vi "Wait Until Not Busy.vi"(6 "chip select  (1st chip)":enum16{"1st chip", "2nd chip"}(ring), 8 "error in (no error)":errorcluster, 11 "LCD in":u32) -> (0 "error out":errorcluster, 3 "LCD out":u32)   [LabVIEW 2015, in "HD44780 FPGA.lvlib"]
uses:
  <vilib>/EmbeddedDisplay/Hitachi HD44780/FPGA/HD44780 FPGA.lvlib
  <vilib>/EmbeddedDisplay/Hitachi HD44780/Common/HD44780 Common.lvlib
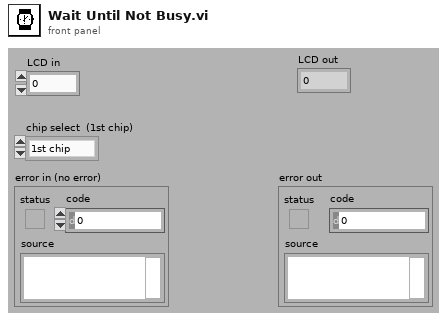
[diagram p1: front panel]
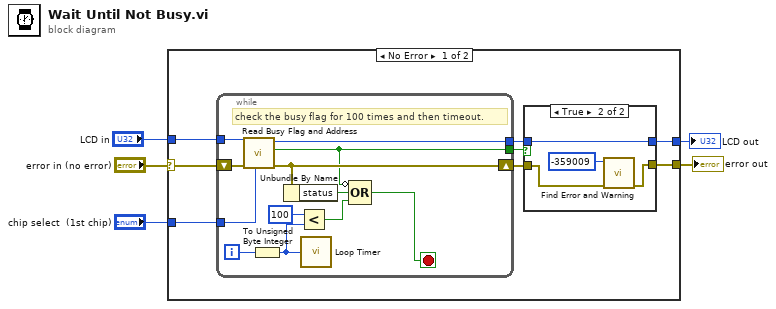
[diagram p0: block diagram]
diagram:
  n1 = case shown="No Error" "error in (no error)" {
    selector: "error in (no error)" -> [w9 w33]
    tunnel: [w12 w33] -> w4
    tunnel: "chip select  (1st chip)" -> [w10 _]
    tunnel: "LCD in" -> [w8 w32]
    tunnel: [w7 w32] -> w1
    frame No Error {
      n2 = while {
        shift-right: [w23] -> w11
        shift-left: w9 -> [w24]
        tunnel: w10 -> [w14]
        tunnel: [w22] -> w13
        tunnel: w8 -> [w21]
        tunnel: [w20] -> w6
        i -> [w18]
        stop <- w19 stop-if-true
        # "check the busy flag for 100 times and then timeout."
        n3 = call <vilib>:"Read Busy Flag and Address.vi"("chip select (1st chip)"=w14, "error in (no error)"=w24, "LCD in"=w21) -> ("error out"=w23:errorcluster, "busy flag"=w22:bool, "LCD out"=w20:u32)  [unwired: 5 in, 1 out]
        n4 = To Unsigned Byte Integer(number=w18) -> (unsigned 8bit integer=w15:u8)
        n5 = Unbundle By Name(w23) -> ("status"=w25:bool)
        n6 = Less?(x=u8 100, y=w15) -> (x < y?=w16:bool)
        n7 = call "Loop Timer"("Count(mSec)"=w15) -> ()  [unwired: 1 out]
        n8 = Compound Arithmetic op=OR(invert w22, w25, w16) -> (w19:bool)
      }
      n9 = case shown="True" w13 {
        tunnel: [w27 w28] -> w12
        tunnel: w11 -> [w27 w29]
        tunnel: [w26 w31] -> w7
        tunnel: w6 -> [w26 w31]
        frame False {
        }
        frame True {
          n10 = call <vilib>:"Find Error and Warning.vi"("error in (no error)"=w29, "error code"=-359009) -> ("error out"=w28:errorcluster)  [unwired: 9 in]
        }
      }
    }
    frame Error {
    }
  }
  "error out" <- w4
  "LCD out" <- w1
